vi "Ex 1 - Avoid Nested Loops.vi"() -> ()   [LabVIEW 2019]
uses:
  53bea0e7-c98c-4da3-80f4-5fafb124b5f4.vi
panel:
  out "Cartesian product":T1(c389)
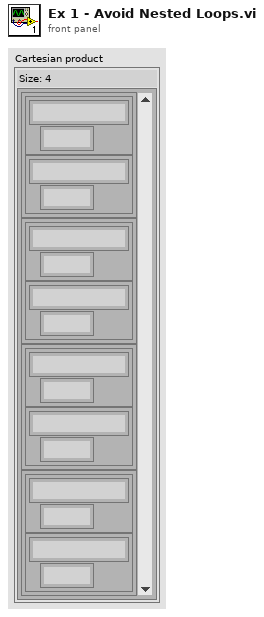
[diagram p1: front panel]
types:
  T1 = set{cluster{cluster{string, i32}, cluster{string, i32}}}
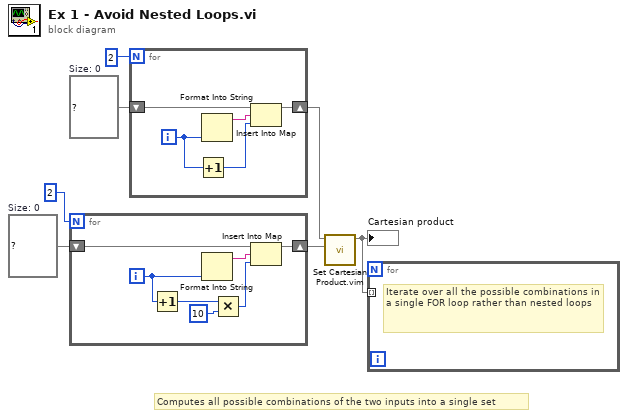
[diagram p0: block diagram]
diagram:
  w4 = map{string, i32} {}  # Size: 0
  w7 = map{string, i32} {}  # Size: 0
  # "Computes all possible combinations of the two inputs into a single set"
  n1 = for {
    N: 2 -> [_]
    shift-right: [w13] -> w2
    shift-left: w4 -> [w14]
    i -> [w11]
    n2 = Increment(x=w11) -> (x+1=w8:i32)
    n3 = Format Into String(w11) -> (resulting string=w12:string)  [unwired: 3 in, 1 out]
    n4 = Multiply(x=w8, y=10) -> (x*y=w9:i32)
    n5 = Insert Into Map(map in=w14, key=w12, value=w9) -> (map out=w13:map{string, i32})  [unwired: 2 out]
  }
  n6 = for {
    N: 2 -> [_]
    shift-right: [w18] -> w3
    shift-left: w7 -> [w19]
    i -> [w16]
    n7 = Increment(x=w16) -> (x+1=w15:i32)
    n8 = Format Into String(w16) -> (resulting string=w17:string)  [unwired: 3 in, 1 out]
    n9 = Insert Into Map(map in=w19, key=w17, value=w15) -> (map out=w18:map{string, i32})  [unwired: 2 out]
  }
  n10 = call "Set Cartesian Product.vim"("set 2"=w2, "set 1"=w3) -> ("Cartesian product"=w1:T1)  [unwired: 9 in]
  "Cartesian product" <- w1
  n11 = for {
    tunnel: w1 -> [_] mode=indexing
    # "Iterate over all the possible combinations in a single FOR loop rather than nested loops"
  }
